vi "Main.vi"() -> ()   [LabVIEW 2020, in "NoCodeEngine.lvlib"]
uses:
  NoCodeEngine.lvlib
  <vilib>/Utility/Data Type/NI_Data Type.lvlib
panel:
  out "Log":string
  in  "stop":bool
  in  "VI Path":path
  # "Set this path to the location of the Simple Controls GUI.vi file before running this VI.\nYou can drag and drop the VI listing in the project onto the path control."
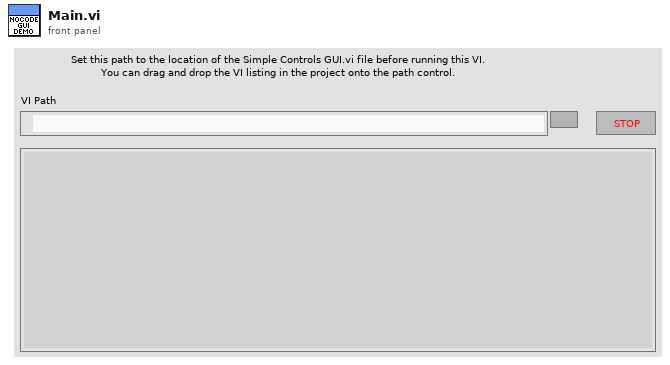
[diagram p1: front panel]
types:
  T1 = enum32{"Invalid", "Standard", "Closed", "Hidden", "Minimized", "Maximized"}
  T2 = typedef "NI_Data Type.lvlib/Data Type.ctl" = enum8{"Invalid Type", "Void", "I8", "I16", "I32", "I64", "U8", "U16", "U32", "U64", "Single Float", "Double Float", "Extended Float", "Single Complex", "Double Complex", "Extended Complex", "Enum U8", "Enum U16", "Enum U32", "Enum U64", "Single Float With Unit", "Double Float With Unit", "Extended Float With Unit", "Single Complex with Unit", "Double Complex with Unit", "Extended Complex with Unit", "Boolean", "String", "Path", "Picture", "Tag", "Array", "Cluster", "Variant", "LV Variant", "Waveform", "Timestamp", "Digital Waveform", "Digital Data", "ExpressData", "Refnum", "External Data", "VI", "Poly VI", "LabVIEW Class Instance", "Fixed Point", "Set Collection", "Map Collection"}
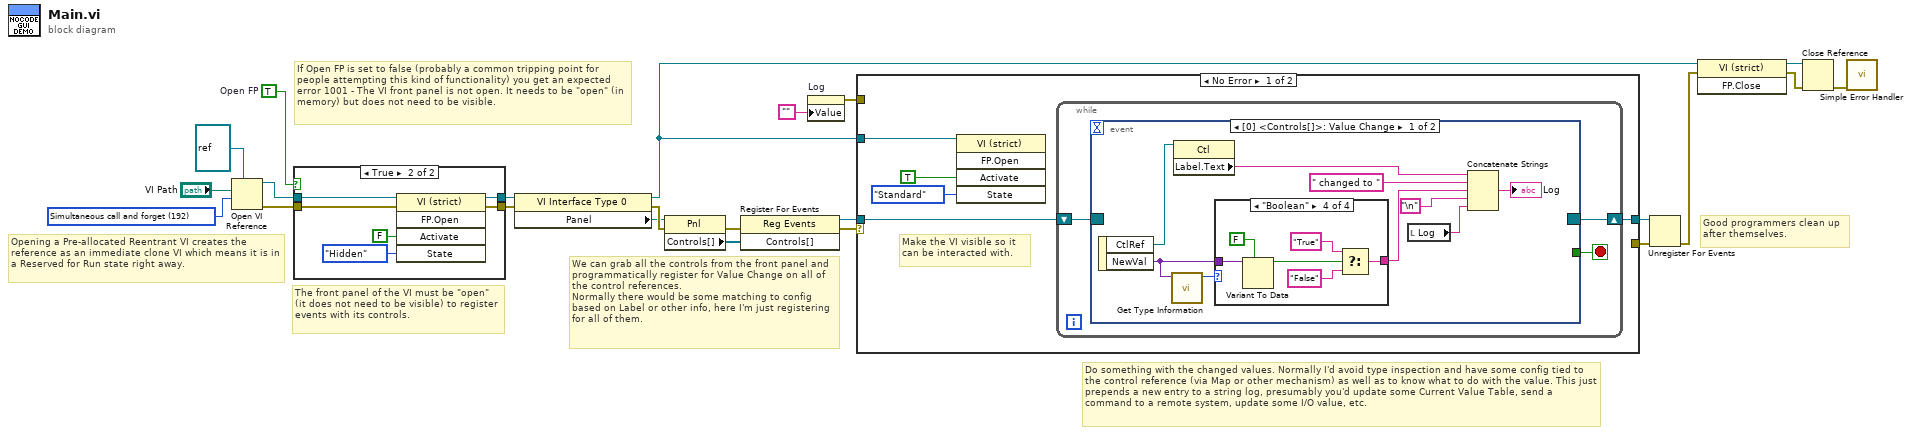
[diagram p0: block diagram]
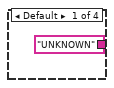
[diagram p3: hidden frame]
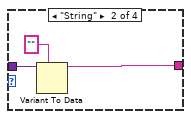
[diagram p4: hidden frame]
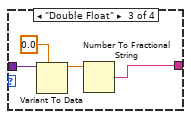
[diagram p5: hidden frame]
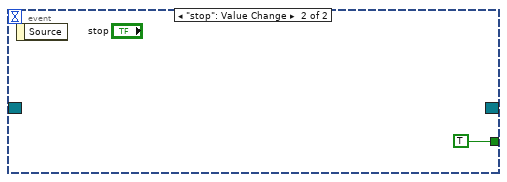
[diagram p6: hidden frame]
diagram:
  w17 = 192 items=["Record modifications"=1, "Open templates for editing"=2, "Prompt user to save"=4, "Prepare for reentrant run"=8, "Prompt to find missing subVIs"=16, "Hide loading dialog box"=32, "Enable simultaneous calls"=64, "Prepare to call and forget"=128, "Simultaneous call and forget"=192, "Prepare to call and collect"=256, "Simultaneous call and collect"=320]
  w21 = TRUE  # Open FP
  # "If Open FP is set to false (probably a common tripping point for people attempting this kind of functionality) you get an expected error 1001 - The VI front panel is not open. It needs to be \"open\" (in memory) but does not need to be visible."
  # "Good programmers clean up after themselves."
  # "Do something with the changed values. Normally I'd avoid type inspection and have some config tied to the control reference (via Map or other mechanism) as well as to know what to do with the value. This just prepends a new entry to a string log, presumably you'd update some Current Value Table, send a command to a remote system, update some I/O value, etc."
  # "We can grab all the controls from the front panel and programmatically register for Value Change on all of the control references.\nNormally there would be some matching to config based on Label or other info, here I'm just registering for all of them."
  # "The front panel of the VI must be \"open\" (it does not need to be visible) to register events with its controls."
  # "Opening a Pre-allocated Reentrant VI creates the reference as an immediate clone VI which means it is in a Reserved for Run state right away."
  n1 = Open VI Reference(type specifier VI Refnum (for type only)=refnum<vi> refnum, vi path="VI Path", options=w17) -> (vi reference=w20:refnum<vi>, error out=w19:errorcluster)  [unwired: 3 in]
  n2 = case shown="True" w21 {
    tunnel: w19 -> [w24 w31]
    tunnel: w20 -> [w25 w30]
    tunnel: [w25 w27] -> w16
    tunnel: [w24 w26] -> w15
    frame False {
    }
    frame True {
      n3 = invoke class="VI (strict)" method="FP.Open"(reference=w30, error in=w31, "Activate"=FALSE ("Activate?"), "State"=T1."Hidden") -> (reference out=w27:refnum<vi>, error out=w26:errorcluster)  [unwired: 1 in, 3 out]
    }
  }
  n4 = property class="VI Interface Type 0"(reference=w16, error in=w15) -> (reference out=w7:refnum<vi>, error out=w23:errorcluster, "Panel"=w14:refnum<vi>)
  n5 = property class="Pnl"(reference=w14, error in=w23) -> (error out=w12:errorcluster, "Controls[]"=w13:refnum<vi>[])  [unwired: 1 out]
  n6 = register-events(error in=w12, w13) -> (reference out=w11:refnum<event-registration>, error out=w9:errorcluster)  [unwired: 1 in]
  n7 = property on="Log" class="Str"("Value"="") -> (error out=w2:errorcluster)  [unwired: 2 in, 1 out]
  n8 = case shown="No Error" w9 {
    selector: w9 -> [_ w64]
    tunnel: w11 -> [w36 w65]
    tunnel: [w35 w65] -> w10
    tunnel: [_ w64] -> w8
    tunnel: w7 -> [w34 _]
    tunnel: w2 -> [_ _]
    frame No Error {
      # "Make the VI visible so it can be interacted with."
      n9 = invoke class="VI (strict)" method="FP.Open"(reference=w34, "Activate"=TRUE ("Activate?"), "State"=T1."Standard") -> ()  [unwired: 2 in, 5 out]
      n10 = while {
        shift-right: [w38] -> w35
        shift-left: w36 -> [w39]
        stop <- w37 stop-if-true
        n11 = event shown="[0] <Controls[]>: Value Change" {
          selector: w39 -> [_ _]
          dyn-events: [_ _] -> w38
          timeout: _ -> [_ _]
          tunnel: [_ TRUE] -> w37
          event Value Change {
            n12 = event-data() -> ("CtlRef"=w48:refnum<vi>, "NewVal"=w47:variant)  [unwired: 1 in]
            n13 = call <vilib>:"Get Type Information.vi"("variant"=w47) -> ("type"=w46:T2)  [unwired: 6 in, 4 out]
            n14 = property class="Ctl"(reference=w48) -> ("Label.Text"=w45:string)  [unwired: 1 in, 2 out]
            n15 = case shown="\"Boolean\"" w46 {
              tunnel: w47 -> [_ w52 w56 w62]
              tunnel: ["UNKNOWN" w50 w53 w57] -> w43
              frame Default {
              }
              frame "String" {
                n16 = Variant To Data(type="", Variant=w52) -> (data=w50:string)  [unwired: 1 in, 1 out]
              }
              frame "Double Float" {
                n17 = Variant To Data(type=0.0, Variant=w56) -> (data=w54:dbl)  [unwired: 1 in, 1 out]
                n18 = Number To Fractional String(number=w54) -> (F-format string=w53:string)  [unwired: 3 in]
              }
              frame "Boolean" {
                n19 = Variant To Data(type=FALSE, Variant=w62) -> (data=w60:bool)  [unwired: 1 in, 1 out]
                n20 = Select(t="True", s=w60, f="False") -> (s? t:f=w57:string)
              }
            }
            n21 = local read "Log"() -> (w41:string)
            n22 = Concatenate Strings(w45, " changed to " ("string"), w43, "\n", w41) -> (→"Log":string)
          }
          event "stop": Value Change {
            n23 = event-data() -> ()  [unwired: 1 in, 1 out]
          }
        }
      }
    }
    frame Error {
    }
  }
  n24 = Unregister For Events(event registration refnum=w10, error in=w8) -> (error out=w4:errorcluster)
  n25 = invoke class="VI (strict)" method="FP.Close"(reference=w7, error in=w4) -> (reference out=w5:refnum<vi>, error out=w3:errorcluster)  [unwired: 1 in, 1 out]
  n26 = Close Reference(reference=w5, error in (no error)=w3) -> (error out=w6:errorcluster)
  n27 = call <vilib>:"Simple Error Handler.vi"("error in (no error)"=w6) -> ()  [unwired: 4 in, 5 out]
